vi "Set_Parameter_Instrument (Json).vi"(8 "error in (no error)":errorcluster caption="entrée d'erreur (pas d'erreur)", 10 "Parameter (Json)":string, 11 "Read_Led_Analyser en entrée":refnum<class "Read_Led_Analyser.lvclass">) -> (0 "error out":errorcluster caption="sortie d'erreur", 3 "Read_Led_Analyser en sortie":refnum<class "Read_Led_Analyser.lvclass">)   [LabVIEW 2020, in "Library Test.lvlib" / "Read_Led_Analyser.lvclass"]
uses:
  Read_Led_Analyser.lvclass
  C:/Users/ngarcin/OneDrive - Altyor/Standard TB/Class/Test/Test (Default)/Test (Default).lvclass
  Commun VI/TypeDef/Commande Led_Analyser/Parametre LED analyser.ctl
  LED Analyser/Class Led Analyser (Default)/Class LED Analyser (Default).lvclass
  JSON API/JSON Value/Set from JSON string.vi
  JSON API/Variant JSON/Variant to JSON.vi
  JSON API/JSON Value/Get Item by name array.vi
  Instrument/Instrument (Default)/Class Instrument (Default).lvclass
  JSON API/JSON Value/JSON Value.lvclass
  Read_Led_Analyser.lvclass/Read_Led_Analyser.ctl
  JSON API/Variant JSON/Variant JSON.lvlib
  JSON API/Get Polymorphic/JSON GetSet.lvlib
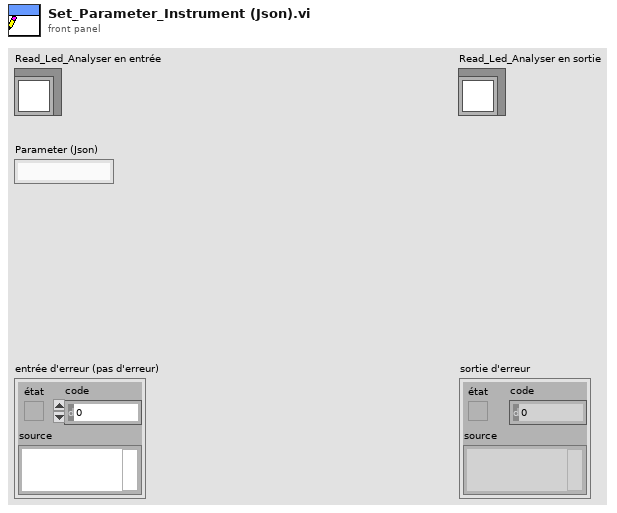
[diagram p1: front panel]
types:
  T1 = typedef "Parametre LED analyser.ctl" = cluster{"Device @":string, "Channel":u16, "LED Analyser":refnum<class "Class LED Analyser (Default).lvclass">}
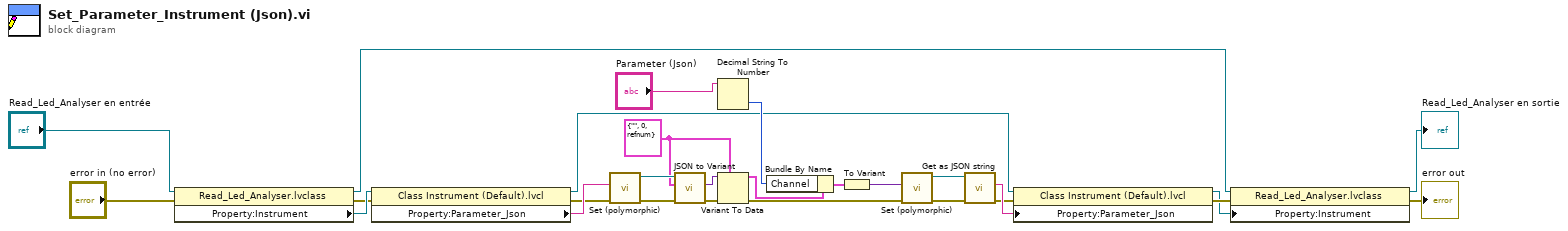
[diagram p0: block diagram]
diagram:
  w23 = T1 {"Device @"="", "Channel"=0, "LED Analyser"=refnum} ("Parameter")
  n1 = property class="Read_Led_Analyser.lvclass"(reference="Read_Led_Analyser en entrée", error in="error in (no error)") -> (reference out=w5:refnum<class "Read_Led_Analyser.lvclass">, error out=w18:errorcluster, "Property:Instrument"=w19:refnum<class "Class Instrument (Default).lvclass">)
  n2 = property class="Class Instrument (Default).lvcl"(reference=w19, error in=w18) -> (reference out=w13:refnum<class "Class Instrument (Default).lvclass">, error out=w16:errorcluster, "Property:Parameter_Json"=w17:string)
  n3 = call-poly "Set (polymorphic).vi"("error in (no error)"=w16, "JSON stream"=w17) -> ("error out"=w25:errorcluster, "JSON Value out"=w27:refnum<class "JSON Value.lvclass">)  [unwired: 7 in, 1 out]
  n4 = call "JSON to Variant.vi"("error in (no error)"=w25, "Variant (Data Type)"=w23, "JSON Value"=w27) -> ("error out"=w26:errorcluster, "Variant out"=w24:variant)  [unwired: 7 in]
  n5 = Decimal String To Number(string="Parameter (Json)") -> (number=w14:i32)  [unwired: 2 in, 1 out]
  n6 = Variant To Data(error in=w26, type=w23, Variant=w24) -> (data=w15:T1, error out=w2:errorcluster)
  n7 = Bundle By Name(cluster=w15, "Channel"=w14) -> (w9:T1)
  n8 = To Variant(anything=w9) -> (Variant=w12:variant)
  n9 = call-poly "Set (polymorphic).vi"("error in (no error)"=w2, "Variant"=w12) -> ("error out"=w10:errorcluster, "JSON Value out"=w11:refnum<class "JSON Value.lvclass">)  [unwired: 8 in]
  n10 = call "Get as JSON string.vi"("error in (no error)"=w10, "JSON Value in"=w11) -> ("error out"=w1:errorcluster, "<JSON>"=w8:string)  [unwired: 8 in]
  n11 = property class="Class Instrument (Default).lvcl"(reference=w13, error in=w1, "Property:Parameter_Json"=w8) -> (reference out=w6:refnum<class "Class Instrument (Default).lvclass">, error out=w7:errorcluster)
  n12 = property class="Read_Led_Analyser.lvclass"(reference=w5, error in=w7, "Property:Instrument"=w6) -> (reference out=→"Read_Led_Analyser en sortie":refnum<class "Read_Led_Analyser.lvclass">, error out=→"error out":errorcluster)
